vi "Sensor Setting.vi"(8 "error in":errorcluster) -> (0 "error  out":errorcluster)   [LabVIEW 2015]
uses:
  Control Button/Save.ctl
  Control Button/Exit.ctl
  <vilib>/addons/database/Connection.llb/DB Tools Open Connec (String).vi
  Galobal variable_TI.vi
  <vilib>/addons/database/_DB Variant To Data/Database Variant To Data.xnode
  <vilib>/addons/database/NI_Database_API.lvlib
panel:
  out "Actuator2(mm)":dbl format="%0.03f"
  out "Actuator1(mm)":dbl format="%0.03f"
  out "Load(N)":dbl format="%0.03f"
  out "data":string[](array[string])
  in  "String":string
  in  "Setting Data":T1
  out "Model":string
  in  "Model":string(combo)
  in  "Exit":T2
  in  "Save":T3
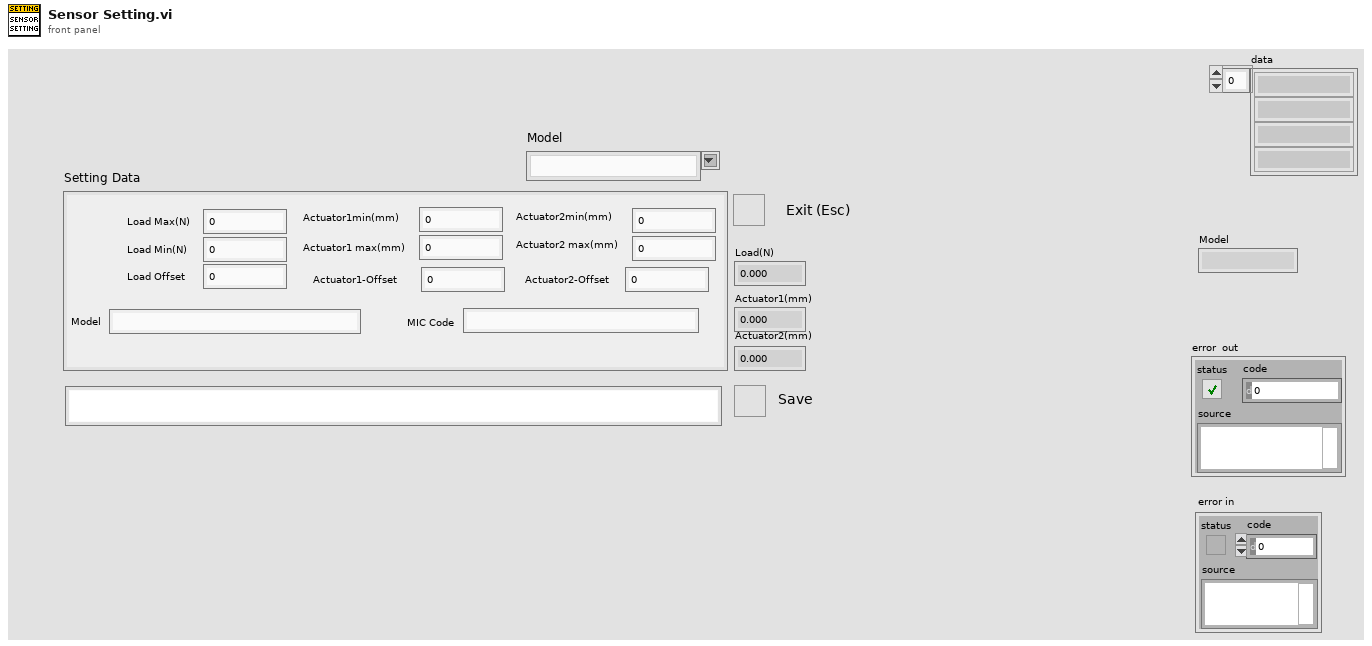
[diagram p1: front panel]
types:
  T1 = cluster{"Load Max(N)":dbl, "Load Min(N)":dbl, "Actuator1 max(mm)":dbl, "Actuator1min(mm)":dbl, "Actuator2 max(mm)":dbl, "Actuator2min(mm)":dbl, "Load Offset":dbl, "Model":string, "MIC Code":string, "Actuator1-Offset":dbl, "Actuator2-Offset":dbl}
  T2 = typedef "Exit.ctl" = bool
  T3 = typedef "Save.ctl" = bool
  T4 = typedef "NI_Database_API.lvlib/Conn ObjectReference.ctl" = refnum<k1>
  T5 = enum16{"Left Button", "Center Button", "Right Button", "Window Close"}
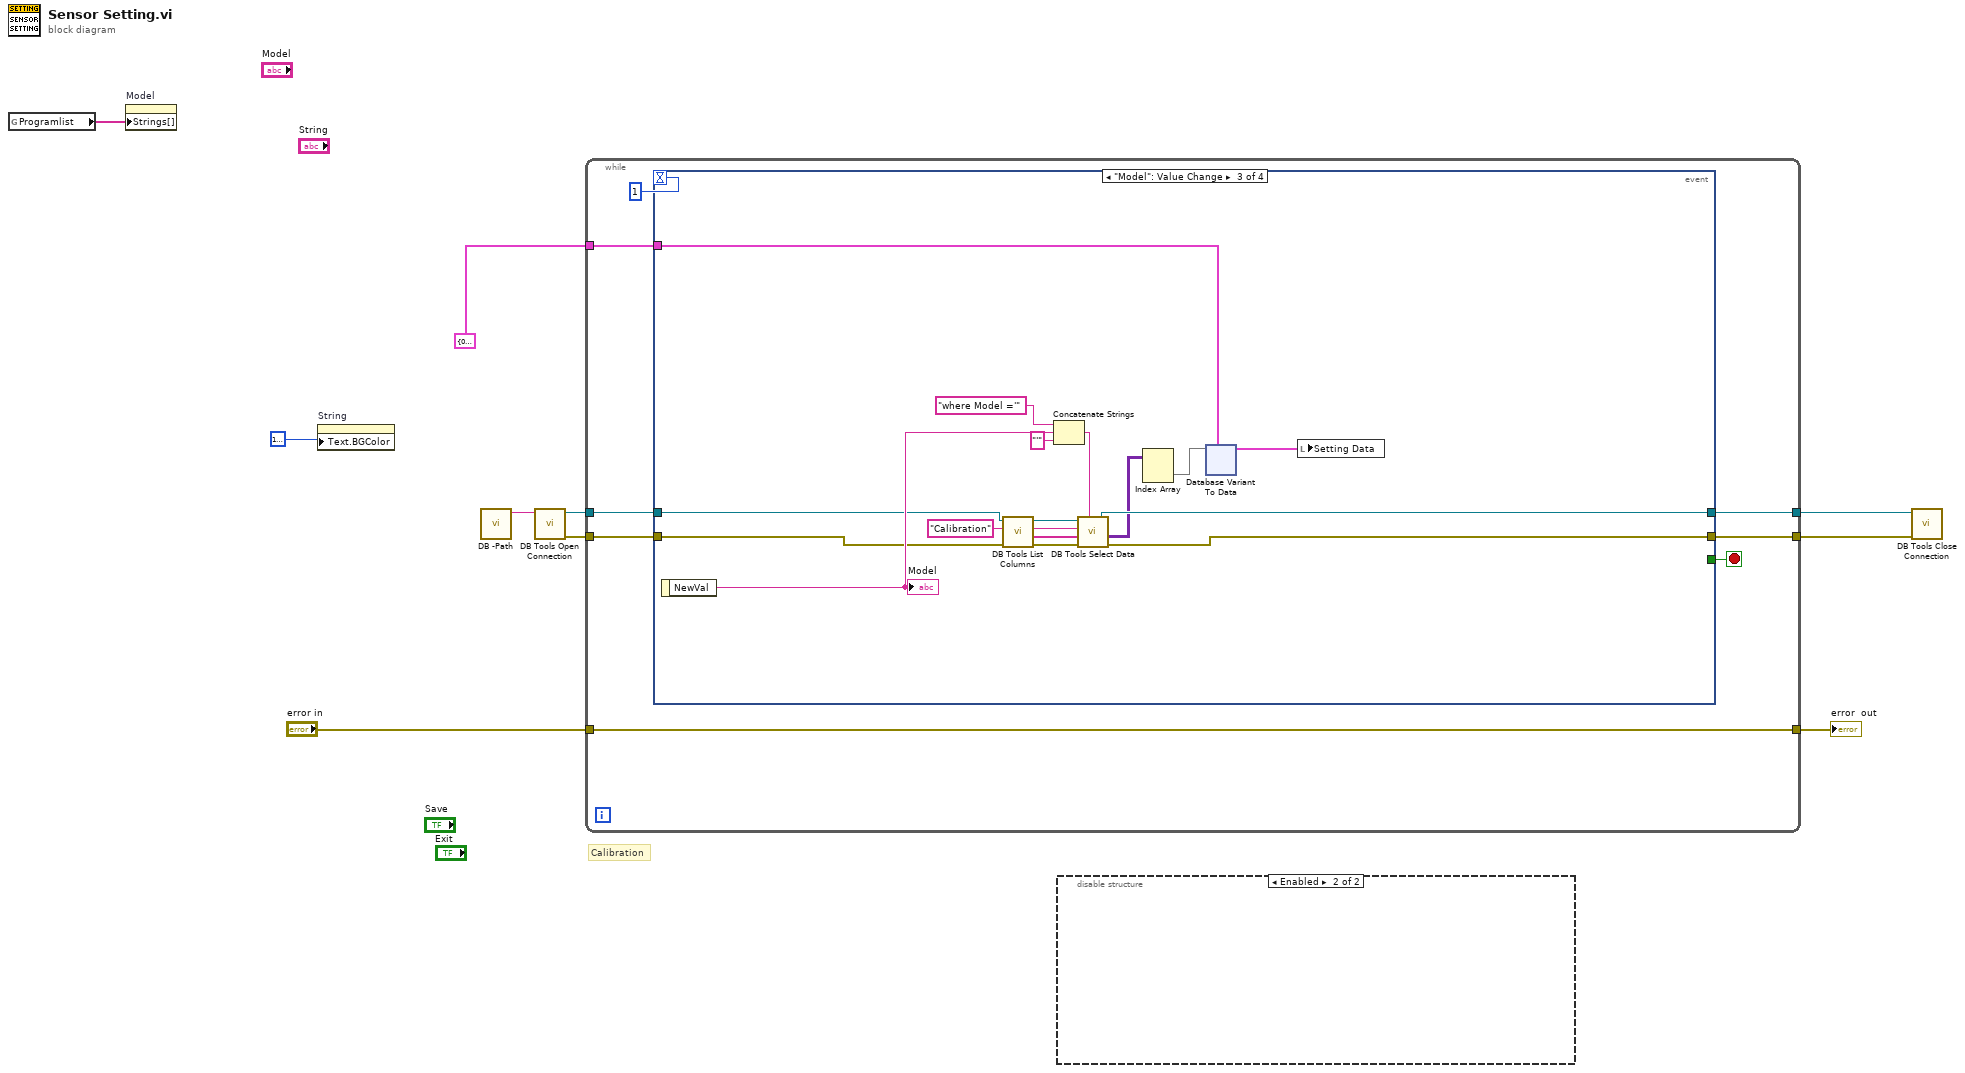
[diagram p0: block diagram]
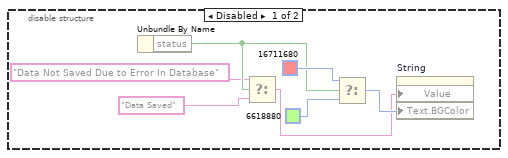
[diagram p2: hidden frame]
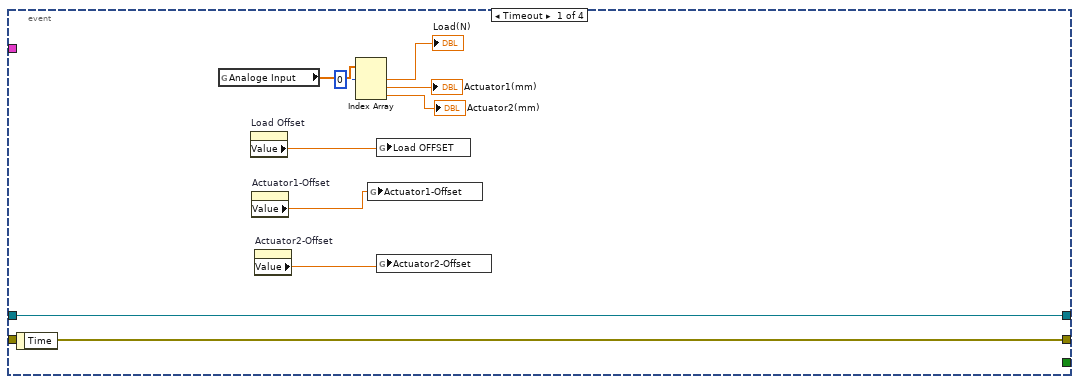
[diagram p3: hidden frame]
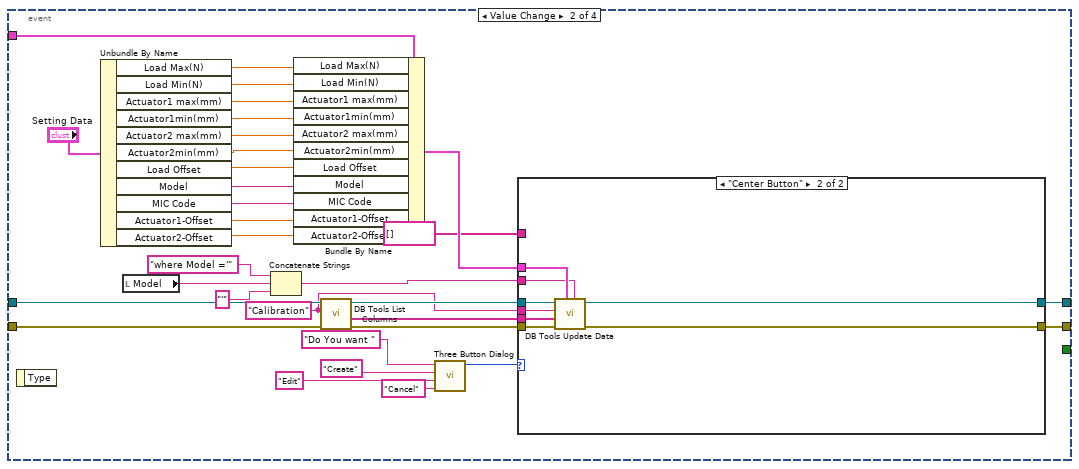
[diagram p4: hidden frame]
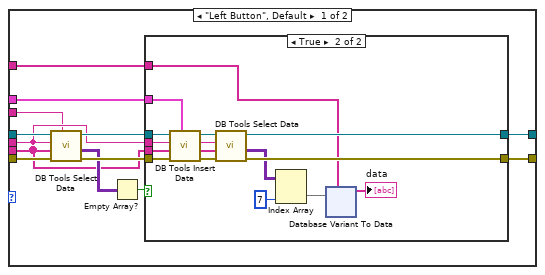
[diagram p5: hidden frame]
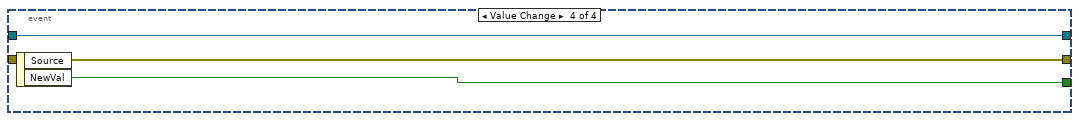
[diagram p7: hidden frame]
diagram:
  # "Calibration"
  n1 = global read "Galobal variable_TI.vi" "Programlist"() -> (w5:string[])
  n2 = property on="Model" class="CmbBox"("Strings[]"=w5) -> ()  [unwired: 2 in, 2 out]
  n3 = property on="String" class="Str"("Text.BGColor"=u32 16777226 ("Color Box")) -> ()  [unwired: 2 in, 2 out]
  n4 = call "DB -Path.vi"() -> ("String"=w10:string)  [unwired: 11 in]
  n5 = call-poly <vilib>:"DB Tools Open Connection.vi"("connection information"=w10) -> ("error out"=w8:errorcluster, "connection reference"=w9:T4)  [unwired: 7 in]
  n6 = while {
    tunnel: w9 -> [w17]
    tunnel: w8 -> [w16]
    tunnel: [w15] -> w7
    tunnel: [w14] -> w6
    tunnel: "error in" -> [w12]
    tunnel: [w12] -> w3
    tunnel: T1 {"Load Max(N)"=0.0, "Load Min(N)"=0.0, "Actuator1 max(mm)"=0.0, "Actuator1min(mm)"=0.0, "Actuator2 max(mm)"=0.0, "Actuator2min(mm)"=0.0, "Load Offset"=0.0, "Model"="", "MIC Code"="", "Actuator1-Offset"=0.0, "Actuator2-Offset"=0.0} ("Setting Data 2") -> [w11]
    stop <- w13 stop-if-true
    n7 = event shown="[2] \"Model\": Value Change" {
      selector: _ -> [_ _ _ _]
      dyn-events: _ -> [_ _ _ _]
      timeout: 1 -> [_ _ _ _]
      tunnel: w17 -> [w28 w58 w143 w498]
      tunnel: w16 -> [w27 w57 w142 w499]
      tunnel: [w28 w55 w141 w498] -> w15
      tunnel: [w27 w49 w140 w499] -> w14
      tunnel: [_ _ _ w497] -> w13
      tunnel: w11 -> [_ w50 w137 _]
      event Timeout {
        n8 = event-data() -> ()  [unwired: 1 in, 1 out]
        n9 = global read "Galobal variable_TI.vi" "Analoge Input"() -> (w25:dbl[])
        n10 = property on="Load Offset" class="DigNum (strict)"() -> ("Value"=w26:dbl)  [unwired: 2 in, 2 out]
        n11 = property on="Actuator1-Offset" class="DigNum (strict)"() -> ("Value"=w20:dbl)  [unwired: 2 in, 2 out]
        n12 = property on="Actuator2-Offset" class="DigNum (strict)"() -> ("Value"=w19:dbl)  [unwired: 2 in, 2 out]
        n13 = Index Array(array=w25, index #1=0 ("index")) -> (element #1=→"Load(N)":dbl, element #2=→"Actuator1(mm)":dbl, element #3=→"Actuator2(mm)":dbl)  [unwired: 2 in]
        n14 = global write "Galobal variable_TI.vi" "Actuator1-Offset"(w20) -> ()
        n15 = global write "Galobal variable_TI.vi" "Load OFFSET"(w26) -> ()
        n16 = global write "Galobal variable_TI.vi" "Actuator2-Offset"(w19) -> ()
      }
      event Value Change {
        w52 = "Calibration" ("table")
        n17 = event-data() -> ()  [unwired: 1 in, 1 out]
        n18 = Unbundle By Name("Setting Data") -> ("Load Max(N)"=w47:dbl, "Load Min(N)"=w46:dbl, "Actuator1 max(mm)"=w45:dbl, "Actuator1min(mm)"=w44:dbl, "Actuator2 max(mm)"=w43:dbl, "Actuator2min(mm)"=w42:dbl, "Load Offset"=w41:dbl, "Model"=w39:string, "MIC Code"=w40:string, "Actuator1-Offset"=w30:dbl, "Actuator2-Offset"=w29:dbl)
        n19 = local read "Model"() -> (w51:string)
        n20 = Concatenate Strings("where Model ='" ("string"), w51, "'" ("string")) -> (w38:string)
        n21 = Bundle By Name(cluster=w50, "Load Max(N)"=w47, "Load Min(N)"=w46, "Actuator1 max(mm)"=w45, "Actuator1min(mm)"=w44, "Actuator2 max(mm)"=w43, "Actuator2min(mm)"=w42, "Load Offset"=w41, "Model"=w39, "MIC Code"=w40, "Actuator1-Offset"=w30, "Actuator2-Offset"=w29) -> (w32:T1)
        n22 = call <vilib>:"DB Tools List Columns.vi"("error in (no error)"=w57, "table"=w52, "connection reference"=w58) -> ("error out"=w60:errorcluster, "columns"=w56:string[], "connection reference out"=w59:T4)  [unwired: 1 in, 1 out]
        n23 = call <vilib>:"Three Button Dialog.vi"("Right Button Text (\"Cancel\")"="Cancel" ("Right Button Text (\"Cancel\")"), "Center Button Text (\"No\")"="Edit" ("Left Button Text (\"Yes\")"), "Left Button Text (\"Yes\")"="Create" ("Left Button Text (\"Yes\")"), "message"="Do You want ") -> ("Which Button?"=w37:T5)  [unwired: 7 in]
        n24 = case shown="\"Center Button\"" w37 {
          tunnel: w60 -> [w68 w129]
          tunnel: w59 -> [w69 w130]
          tunnel: w56 -> [w64 w131]
          tunnel: [w67 w135] -> w55
          tunnel: w52 -> [w65 w132]
          tunnel: [w66 w133] -> w49
          tunnel: w38 -> [w62 w128]
          tunnel: w32 -> [w63 w134]
          tunnel: string[] [] -> [w61 _]
          frame "Left Button", Default {
            n25 = call <vilib>:"DB Tools Select Data.vi"("condition"=w62, "error in (no error)"=w68, "columns"=w64, "table"=w65, "connection reference"=w69) -> ("error out"=w72:errorcluster, "data"=w71:variant[][], "connection reference out"=w73:T4)  [unwired: 1 in]
            n26 = Empty Array?(array=w71) -> (empty?=w70:bool)
            n27 = case shown="True" w70 {
              tunnel: w72 -> [w74 w89]
              tunnel: [w75 w82] -> w67
              tunnel: [w74 w81] -> w66
              tunnel: w73 -> [w75 w88]
              tunnel: w65 -> [_ w84]
              tunnel: w64 -> [_ w83]
              tunnel: w63 -> [_ w87]
              tunnel: w61 -> [_ w77]
              frame False {
              }
              frame True {
                n28 = call <vilib>:"DB Tools Insert Data.vi"("data"=w87, "error in (no error)"=w89, "columns"=w83, "table"=w84, "connection reference"=w88) -> ("error out"=w85:errorcluster, "connection reference out"=w86:T4)  [unwired: 5 in]
                n29 = call <vilib>:"DB Tools Select Data.vi"("error in (no error)"=w85, "columns"=w83, "table"=w84, "connection reference"=w86) -> ("error out"=w81:errorcluster, "data"=w80:variant[][], "connection reference out"=w82:T4)  [unwired: 2 in]
                n30 = Index Array(array=w80, index (col)=7 ("disabled index (col)")) -> (element=w78:variant[])  [unwired: 1 in]
                n31 = xnode "Database Variant To Data"("database variant"=w78, "type"=w77) -> ("data"=→"data":string[])  [unwired: 1 in, 1 out]
              }
            }
          }
          frame "Center Button" {
            n32 = call <vilib>:"DB Tools Update Data.vi"("condition"=w128, "data"=w134, "error in (no error)"=w129, "columns"=w131, "table"=w132, "connection reference"=w130) -> ("error out"=w133:errorcluster, "connection reference out"=w135:T4)  [unwired: 4 in]
          }
        }
      }
      event "Model": Value Change {
        w145 = "Calibration" ("table")
        n33 = event-data() -> ("NewVal"=w144:string)  [unwired: 1 in]
        "Model" <- w144
        n34 = call <vilib>:"DB Tools List Columns.vi"("error in (no error)"=w142, "table"=w145, "connection reference"=w143) -> ("error out"=w151:errorcluster, "columns"=w149:string[], "connection reference out"=w150:T4)  [unwired: 1 in, 1 out]
        n35 = Concatenate Strings("where Model ='" ("string"), w144, "'" ("string")) -> (w146:string)
        n36 = call <vilib>:"DB Tools Select Data.vi"("condition"=w146, "error in (no error)"=w151, "columns"=w149, "table"=w145, "connection reference"=w150) -> ("error out"=w140:errorcluster, "data"=w139:variant[][], "connection reference out"=w141:T4)  [unwired: 1 in]
        n37 = Index Array(array=w139) -> (element=w138:variant[])  [unwired: 2 in]
        n38 = xnode "Database Variant To Data"("database variant"=w138, "type"=w137) -> ("data"=w136:T1)  [unwired: 1 in, 1 out]
        n39 = local write "Setting Data"(w136) -> ()
      }
      event Value Change {
        n40 = event-data() -> ("NewVal"=w497:T2)  [unwired: 1 in, 1 out]
      }
    }
  }
  "error  out" <- w3
  n41 = disable-structure shown="Enabled" {
    frame Disabled {
      n42 = Unbundle By Name() -> ("status"=w503:bool)  [unwired: 1 in]
      n43 = Select(t="Data Not Saved Due to Error In Database", s=w503, f="Data Saved") -> (s? t:f=w502:string)
      n44 = Select(t=u32 16711680 ("Color Box"), s=w503, f=u32 6618880 ("Color Box")) -> (s? t:f=w506:u32)
      n45 = property on="String" class="Str"("Value"=w502, "Text.BGColor"=w506) -> ()  [unwired: 2 in, 2 out]
    }
    frame Enabled {
    }
  }
  n46 = call <vilib>:"DB Tools Close Connection.vi"("error in (no error)"=w6, "connection reference"=w7) -> ()  [unwired: 5 in, 1 out]
